vi "Main.vi"() -> ()   [LabVIEW 2018]
uses:
  <vilib>/Utility/miscctls.llb/LVPointTypeDef.ctl
panel:
  in  "Open Tube Control VI":bool
  in  "Open Spark Test VI":bool
  in  "Stop":bool
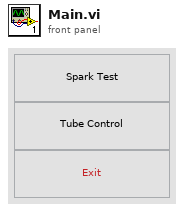
[diagram p1: front panel]
types:
  T1 = typedef "LVPointTypeDef.ctl" = cluster{"Horizontal":i16, "Vertical":i16}
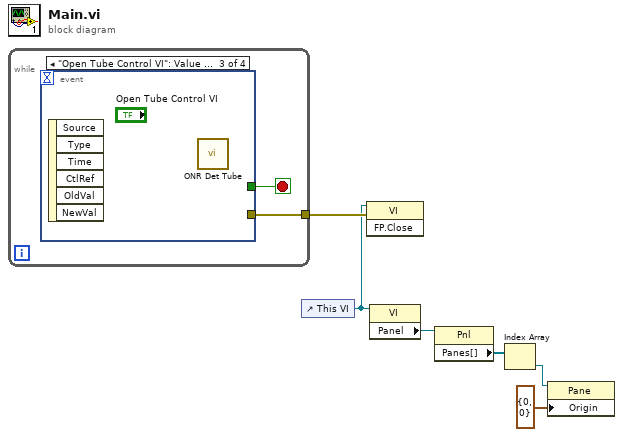
[diagram p0: block diagram]
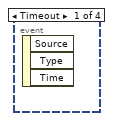
[diagram p2: hidden frame]
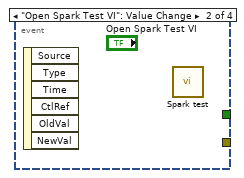
[diagram p3: hidden frame]
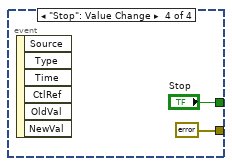
[diagram p4: hidden frame]
diagram:
  n1 = while {
    tunnel: [w7] -> w6
    stop <- w8 stop-if-true
    n2 = event shown="[2] \"Open Tube Control VI\": Value Change" {
      selector: _ -> [_ _ _ _]
      dyn-events: _ -> [_ _ _ _]
      timeout: _ -> [_ _ _ _]
      tunnel: [_ _ _ "Stop"] -> w8
      tunnel: [_ _ _ errorcluster {"status"=FALSE, "code"=0, "source"=""} ("error in (no error)")] -> w7
      event Timeout {
        n3 = event-data() -> ()  [unwired: 1 in, 3 out]
      }
      event "Open Spark Test VI": Value Change {
        n4 = event-data() -> ()  [unwired: 1 in, 6 out]
        n5 = call "Spark test.vi"() -> ()  [unwired: 12 in]
      }
      event "Open Tube Control VI": Value Change {
        n6 = event-data() -> ()  [unwired: 1 in, 6 out]
        n7 = call "ONR Det Tube.vi"() -> ()  [unwired: 12 in]
      }
      event "Stop": Value Change {
        n8 = event-data() -> ()  [unwired: 1 in, 6 out]
      }
    }
  }
  n9 = control-ref of="This VI"() -> (w1:refnum<vi>)
  n10 = invoke class="VI" method="FP.Close"(reference=w1, error in=w6) -> ()  [unwired: 1 in, 3 out]
  n11 = property class="VI"(reference=w1) -> ("Panel"=w2:refnum<vi>)  [unwired: 1 in, 2 out]
  n12 = property class="Pnl"(reference=w2) -> ("Panes[]"=w3:refnum<vi>[])  [unwired: 1 in, 2 out]
  n13 = Index Array(array=w3) -> (element=w4:refnum<vi>)  [unwired: 1 in]
  n14 = property class="Pane"(reference=w4, "Origin"=T1 {"Horizontal"=0, "Vertical"=0}) -> ()  [unwired: 1 in, 2 out]
